vi "VI_Frontmost.vi"(7 "TAG":string, 8 "error in (no error)":errorcluster, 10 "DB Ref":T1, 11 "String":string) -> (0 "error out":errorcluster)   [LabVIEW 2017, in "tagdb-RefMgr Operations.lvlib"]
uses:
  tagdb-RefMgr Operations.lvlib
  <userlib>/_NEVSTOP/TagDB/Typedef/TagDB.ctl
  9d97d59a-d43f-438e-a95f-715b9f62aa35.vi
  9d97d59a-d43f-438e-a95f-715b9f62aa35.vi/1b47866c-8e2d-43a7-815f-8cf18635e5a1.vi
  <userlib>/_NEVSTOP/TagDB/_Support/Error/_Clear Errors.vi
  9d97d59a-d43f-438e-a95f-715b9f62aa35.vi/1b47866c-8e2d-43a7-815f-8cf18635e5a1.vi/29b2ea6d-6d7f-4e4a-ad31-a5cb760462c7.vi
  <userlib>/_NEVSTOP/TagDB/API/TagDB-Status.vi
  <userlib>/_NEVSTOP/TagDB/_Support/DataAccess/_NameCacher.vi
  <userlib>/_NEVSTOP/TagDB/_Support/Change Detector/TagDB dbChanged.vi
  <userlib>/_NEVSTOP/TagDB/_Support/DataAccess/TagDB Ref to DVR.vi
  <userlib>/_NEVSTOP/TagDB/_Support/Error/_[error50000]Invalid DB REF.vi
  <userlib>/_NEVSTOP/TagDB/_Support/URL/TRIM-BOTH-SPACE.vi
  <userlib>/_NEVSTOP/TagDB/_Support/Error/_[error50002]Invalid DataType.vi
  <userlib>/_OpenG.lib/string/string.llb/Trim Whitespace__ogtk.vi
  <userlib>/_OpenG.lib/string/string.llb/Trim Whitespace (String)__ogtk.vi
  <userlib>/_NEVSTOP/TagDB/TagDB.lvlib
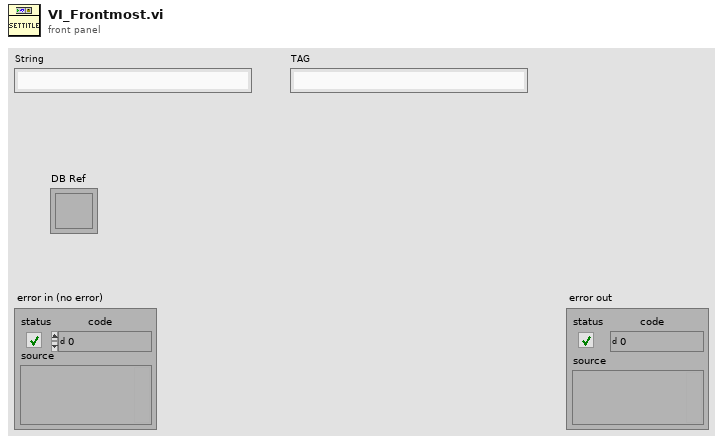
[diagram p1: front panel]
types:
  T1 = typedef "TagDB.lvlib/TagDB.ctl" = refnum<k1>
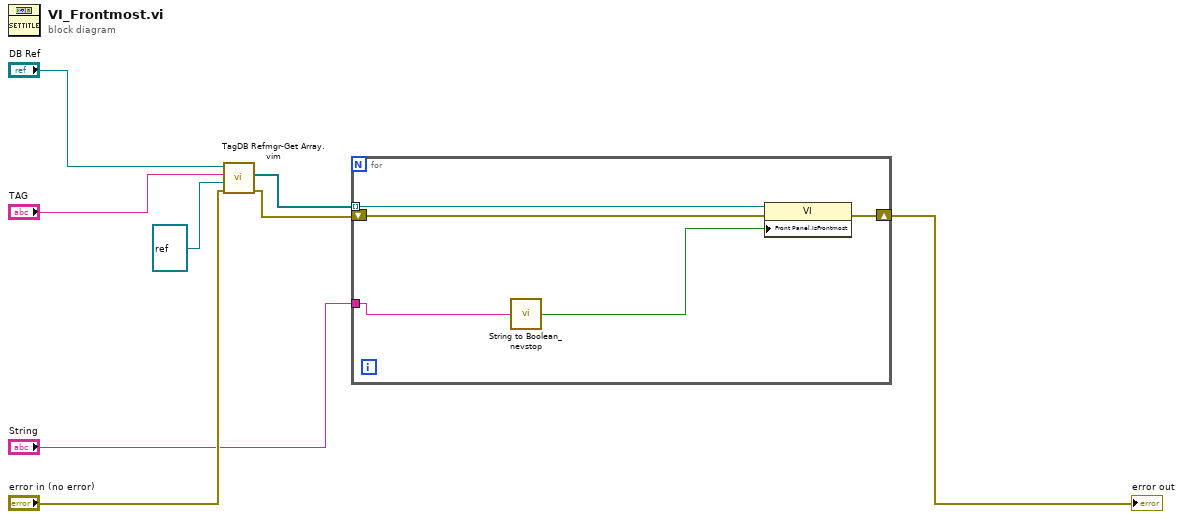
[diagram p0: block diagram]
diagram:
  n1 = call "TagDB Refmgr-Get Array.vim"("error in (no error)"="error in (no error)", "Type"=refnum<vi> refnum ("Current VI Reference"), "RegExp"="TAG", "DB Ref"="DB Ref") -> ("error out"=w3:errorcluster, "References"=w8:refnum<vi>[])  [unwired: 4 in, 2 out]
  n2 = for {
    tunnel: w8 -> [w13] mode=indexing
    shift-right: [w12] -> w2
    shift-left: w3 -> [w11]
    tunnel: "String" -> [w10]
    n3 = call <userlib>:"String to Boolean_nevstop.vi"("String"=w10) -> ("Boolean"=w9:bool)  [unwired: 3 in]
    n4 = property class="VI"(reference=w13, error in=w11, "Front Panel.IsFrontmost"=w9) -> (error out=w12:errorcluster)  [unwired: 1 out]
  }
  "error out" <- w2
